vi "RectEmptyFloat-lv.vi"(1 "R":T1) -> (0 "R is empty?":bool)   [LabVIEW 2024, in "SDL3.lvlib" / "Rect.lvlib"]
doc: "<B>LV Implementation</B>\nSince the SDL function is inlined, we can't access in the shared library. So it's a LabVIEW implementation of the feature.\n\n<B>Summary</B>\nDetermine whether a floating point rectangle can contain any point.\n\n<B>Remarks</B>\nA rectangle is considered \"empty\" for this function if r is NULL, or if r's width and/or height are <= 0."
uses:
  Rect.lvlib
  FRect--cluster.ctl
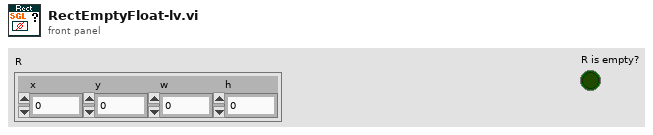
[diagram p1: front panel]
types:
  T1 = typedef "SDL3.lvlib/Rect.lvlib/FRect--cluster.ctl" = cluster{"x":sgl, "y":sgl, "w":sgl, "h":sgl}
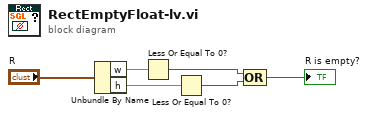
[diagram p0: block diagram]
diagram:
  n1 = Unbundle By Name("R") -> ("w"=w4:sgl, "h"=w3:sgl)
  n2 = Less Or Equal To 0?(x=w4) -> (x <= 0?=w2:bool)
  n3 = Less Or Equal To 0?(x=w3) -> (x <= 0?=w1:bool)
  n4 = Compound Arithmetic op=OR(w2, w1) -> (→"R is empty?":bool)
